vi "CLT_Test State Mach.vi"(6 "Tolerance":dbl, 7 "Pump CtlRef In":T1, 8 "Max Fill in":dbl, 9 "Level PV":dbl, 10 "Level SP":dbl, 11 "TEST STATUS In":T2(ring)) -> (1 "SP out":dbl, 3 "TEST STATUS Out":T2(ring))   [LabVIEW 2024]
doc: "The \"Run Test\" button selects between MANUAL adjustment of Set Point (SP) by the user or AUTO mode, where:\n1. Start, initial state drains until the tank is empty\n2. Filling, Auto set of SP to Max Fill Inches (or recipie)\n3. FULL Pause when full\n4. Draining Auto set of SP to 0 (or recipie)\n5. EMPTY Paue when empty\n6. Done SP set to 0."
uses:
  Control Definitions/Def PumpCtlRefs.ctl
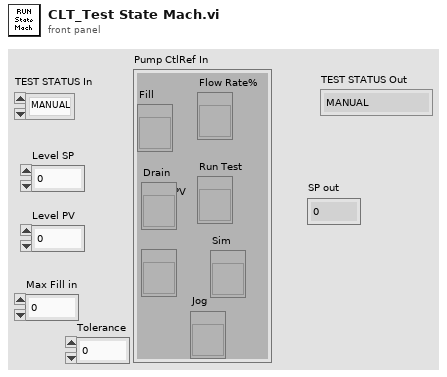
[diagram p1: front panel]
types:
  T1 = typedef "Def PumpCtlRefs.ctl" = cluster{"Fill ":refnum<vi>, "Drain":refnum<vi>, "Level PV":refnum<vi>, "Flow Rate%":refnum<vi>, "Run Test":refnum<vi>, "Sim":refnum<vi>, "Jog":refnum<vi>}
  T2 = enum16{"MANUAL", "Start", "Filling", "FULL", "Draining", "EMPTY", "Done"}
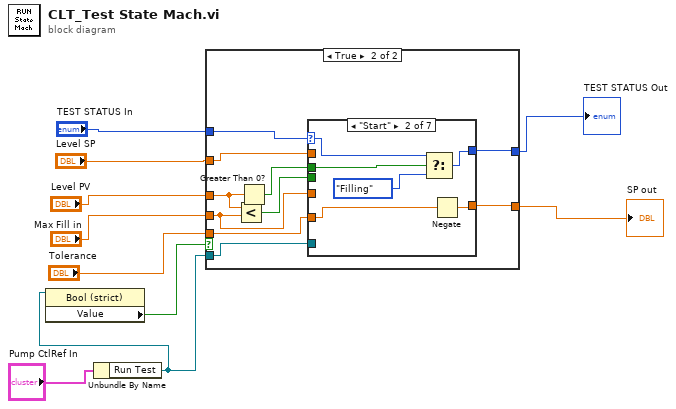
[diagram p0: block diagram]
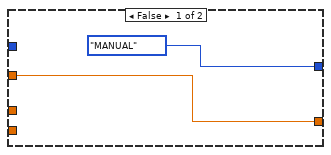
[diagram p2: hidden frame]
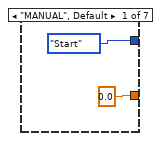
[diagram p3: hidden frame]
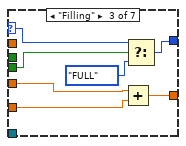
[diagram p4: hidden frame]
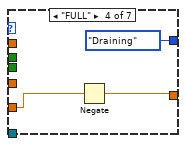
[diagram p5: hidden frame]
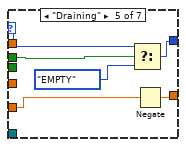
[diagram p6: hidden frame]
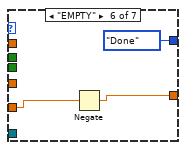
[diagram p7: hidden frame]
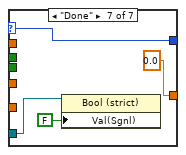
[diagram p8: hidden frame]
diagram:
  n1 = Unbundle By Name("Pump CtlRef In") -> ("Run Test"=w1:refnum<vi>)
  n2 = property class="Bool (strict)"(reference=w1) -> ("Value"=w3:bool)  [unwired: 1 in, 2 out]
  n3 = case shown="True" w3 {
    tunnel: "Level SP" -> [w12 w14]
    tunnel: [w12 w20] -> w5
    tunnel: "TEST STATUS In" -> [_ w17]
    tunnel: "Level PV" -> [_ w21]
    tunnel: [T2."MANUAL" ("TEST STATUS In in") w19] -> w6
    tunnel: "Max Fill in" -> [_ w22]
    tunnel: "Tolerance" -> [_ w15]
    tunnel: w1 -> [_ w13]
    frame False {
    }
    frame True {
      n4 = Less?(x=w21, y=w22) -> (x < y?=w16:bool)
      n5 = Greater Than 0?(x=w21) -> (x > 0?=w18:bool)
      n6 = case shown="\"Start\"" w17 {
        selector: w17 -> [_ w29 w34 _ w44 _ w52]
        tunnel: w22 -> [_ _ w32 _ _ _ _]
        tunnel: [0.0 ("Level SP") w26 w33 w38 w42 w47 0.0 ("Max Inches in")] -> w20
        tunnel: [T2."Start" ("TEST STATUS In in") w27 w36 T2."Draining" ("TEST STATUS In in") w45 T2."Done" ("TEST STATUS In in") w52] -> w19
        tunnel: w18 -> [_ w28 _ _ w43 _ _]
        tunnel: w16 -> [_ _ w35 _ _ _ _]
        tunnel: w15 -> [_ w25 w31 w39 w41 w48 _]
        tunnel: w14 -> [_ _ _ _ _ _ _]
        tunnel: w13 -> [_ _ _ _ _ _ w51]
        frame "MANUAL", Default {
        }
        frame "Start" {
          n7 = Select(t=w29, s=w28, f=T2."Filling" ("TEST STATUS In in")) -> (s? t:f=w27:T2)
          n8 = Negate(x=w25) -> (-x=w26:dbl)
        }
        frame "Filling" {
          n9 = Add(x=w32, y=w31) -> (x+y=w33:dbl)
          n10 = Select(t=w34, s=w35, f=T2."FULL" ("TEST STATUS In in")) -> (s? t:f=w36:T2)
        }
        frame "FULL" {
          n11 = Negate(x=w39) -> (-x=w38:dbl)
        }
        frame "Draining" {
          n12 = Select(t=w44, s=w43, f=T2."EMPTY" ("TEST STATUS In in")) -> (s? t:f=w45:T2)
          n13 = Negate(x=w41) -> (-x=w42:dbl)
        }
        frame "EMPTY" {
          n14 = Negate(x=w48) -> (-x=w47:dbl)
        }
        frame "Done" {
          n15 = property class="Bool (strict)"(reference=w51, "Val(Sgnl)"=FALSE ("Value (Signaling)")) -> ()  [unwired: 1 in, 2 out]
        }
      }
    }
  }
  "TEST STATUS Out" <- w6
  "SP out" <- w5
